vi "KE26XX Factory Pulse Script Usage.vi"(8 "error in":errorcluster, 11 "VISA resource name":refnum<visa-resource-name>) -> (0 "error out":errorcluster, 1 "Buffer Data":string)   [LabVIEW 2012]
doc: "This VI demonstrates how to use the Factory Pulse Script functions within a user script.\n\nThis VI demonstrates the following:\n• How to load and run a user script\n• How to use the Factory Pulse Script functions in a user script\n• How to create and configure a volatile reading buffer in a user script."
uses:
  Keithley 2600 Series.lvlib
panel:
  in  "Script":string="points\t= 10\nsmu = smua\n\t\n-- Configure SMU\nsmu.reset()\n\tsmu.measure.nplc\t\t= 0.001\n\tsmu.measure.autozero\t= smu.AUTOZERO_ONCE\n\tsmu.measure.autorangei\t= smu.AUTORANGE_OFF\n\tsmu.measure.autorangev\t= smu.AUTORANGE_OFF\n\tsmu.source.autorangei\t= smu.AUTORANGE_OFF\n\tsmu.source.autorangev\t= smu.AUTORANGE_OFF\n\tsmu.sense\t\t\t\t= smu.SENSE_LOCAL\n\tsmu.measure.rangei\t\t= 0.01\n\tsmu.measure.rangev\t\t= 20\n\tsmu.source.rangei\t\t= 0.01\n\tsmu.source.rangev\t\t= 20\n\n-- Prepare reading buffer\nmybuf = smu.makebuffer(points)\nmybuf.clear()\nmybuf.appendmode = 1\n\t\nConfigPulseVMeasureI(smu,  0.0, 5.000,  0.01, 1e-3,  1e-3, points, mybuf, 1)\n\t\t\n\tsmu.source.output\t\t= 1\nInitiatePulseTest(1)\n\tsmu.source.output\t\t= 0"
  # "(c) 2008 Keithley Instruments, Inc.  ALL RIGHTS RESERVED."
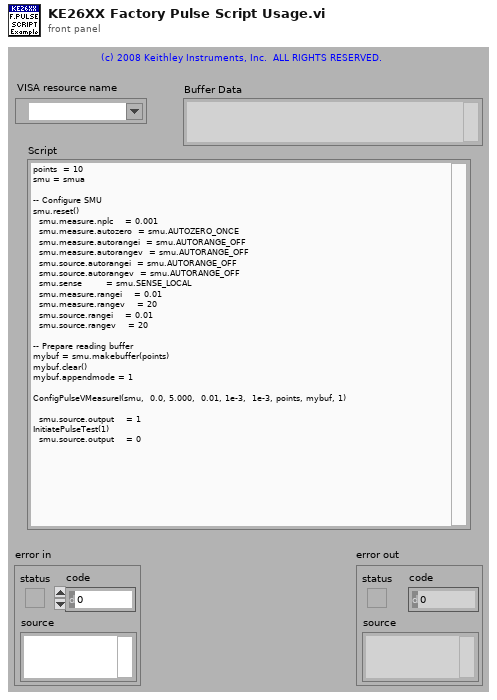
[diagram p1: front panel]
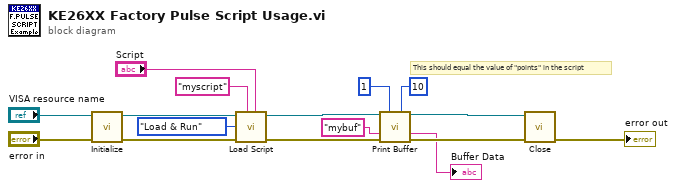
[diagram p0: block diagram]
diagram:
  # "This should equal the value of \"points\" in the script"
  n1 = call "Initialize.vi"("error in (no error)"="error in", "VISA resource name"="VISA resource name") -> ("error out"=w15:errorcluster, "VISA resource name out"=w16:refnum<visa-resource-name>)  [unwired: 4 in, 4 out]
  n2 = call "Load Script.vi"("Script"="Script", "Script Name"="myscript", "error in"=w15, "Load Options (Load)"=enum16{"Load", "Load & Run"}."Load & Run", "VISA resource name"=w16) -> ("error out"=w14:errorcluster, "VISA resource name out"=w11:refnum<visa-resource-name>)  [unwired: 1 in, 4 out]
  n3 = call "Print Buffer.vi"("VISA resource name"=w11, "Start Index (1)"=u32 1, "End Index (1)"=u32 10, "Buffer Name(s)"="mybuf", "error in (no error)"=w14) -> ("VISA resource name out"=w12:refnum<visa-resource-name>, "Buffer Data"=→"Buffer Data":string, "error out"=w13:errorcluster)  [unwired: 2 in, 6 out]
  n4 = call "Close.vi"("error in (no error)"=w13, "VISA resource name"=w12) -> ("error out"=→"error out":errorcluster)  [unwired: 9 out]
